vi "Results.vi"(8 "Error In":errorcluster, 11 "GenAlg_data":T1) -> (0 "Error Out":errorcluster, 2 "Cost":dbl, 3 "MinPoint":dbl[](array[numeric]))   [LabVIEW 2016]
uses:
  TypeDefs/GenAlg_data.ctl
  TypeDefs/basic_config.ctl
  TypeDefs/element.ctl
  TypeDefs/geration_data.ctl
  TypeDefs/selection_data.ctl
  TypeDefs/SimulatedAnnealing_data.ctl
  TypeDefs/multi_eval_data.ctl
  TypeDefs/termination_data.ctl
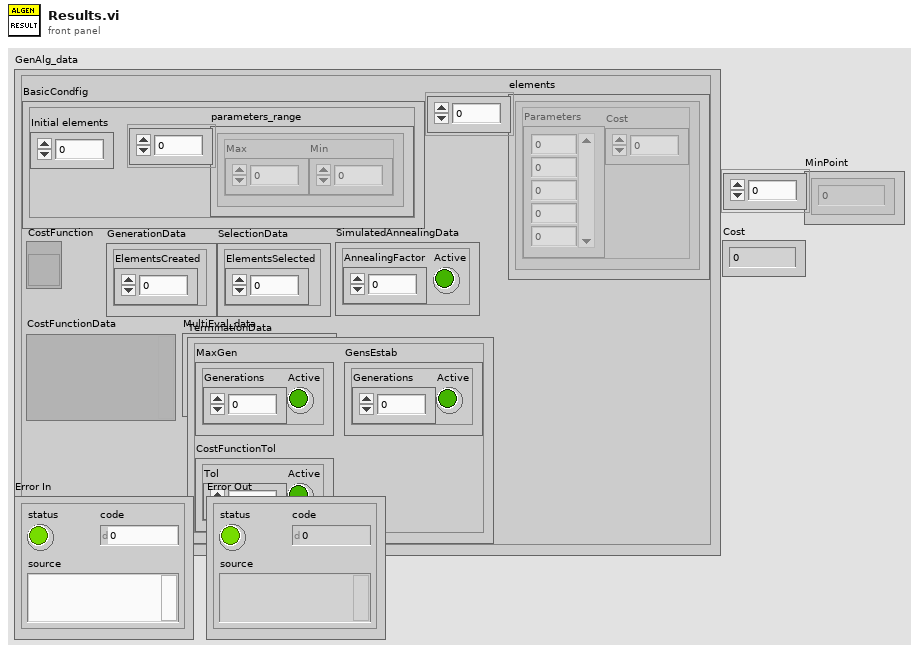
[diagram p1: front panel]
types:
  T1 = typedef "GenAlg_data.ctl" = cluster{"BasicCondfig":T2, "elements":T3[], "CostFunction":refnum<vi>, "GenerationData":T4, "SelectionData":T5, "SimulatedAnnealingData":T6, "CostFunctionData":variant, "MultiEval_data":T7, "TerminationData":T8}
  T2 = typedef "basic_config.ctl" = cluster{"parameters_range":cluster{"Max":dbl, "Min":dbl}[], "Initial elements":i32}
  T3 = typedef "element.ctl" = cluster{"Parameters":dbl[], "Cost":dbl}
  T4 = typedef "geration_data.ctl" = cluster{"ElementsCreated":i32}
  T5 = typedef "selection_data.ctl" = cluster{"ElementsSelected":i32}
  T6 = typedef "SimulatedAnnealing_data.ctl" = cluster{"AnnealingFactor":dbl, "Active":bool}
  T7 = typedef "multi_eval_data.ctl" = cluster{"Active":bool, "MultiEvalFunction":refnum<vi>}
  T8 = typedef "termination_data.ctl" = cluster{"MaxGen":cluster{"Generations":i32, "Active":bool}, "CostFunctionTol":cluster{"Tol":dbl, "Active":bool}, "GensEstab":cluster{"Generations":i32, "Active":bool}}
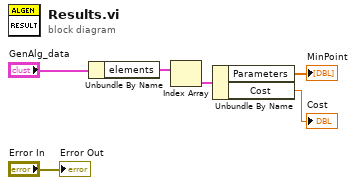
[diagram p0: block diagram]
diagram:
  n1 = Unbundle By Name("GenAlg_data") -> ("elements"=w4:T3[])
  n2 = Index Array(array=w4) -> (element=w3:T3)  [unwired: 1 in]
  n3 = Unbundle By Name(w3) -> ("Parameters"=→"MinPoint":dbl[], "Cost"=→"Cost":dbl)
  "Error Out" <- "Error In"
